vi "数据查询_数据查询.vi"() -> ()   [LabVIEW 2016, in "数据查询.lvlib"]
uses:
  System.Windows.Forms
  <vilib>/Utility/miscctls.llb/LVPointTypeDef.ctl
  <userlib>/_OpenG.lib/array/array.llb/Sort 2D Array (String)__ogtk.vi
  <vilib>/ptbypt/NI_PtbyPt.lvlib
panel:
  in  "数据类型":string(combo)="N"
  out "columns":string[](array[string])
  out "表格":string[][](table)
  in  "剔除异常数据":bool=TRUE
  in  "WebBrowser":refnum<k24>(container)
  in  "列表框":i32(listbox)
  in  "导出":bool
  in  "测量模式":string(combo)="全部数据"
  out "选中数据表":string
  in  "查询":bool
  in  "结束日期":string="2050/01/01"
  in  "起始日期":string="2010/01/01"
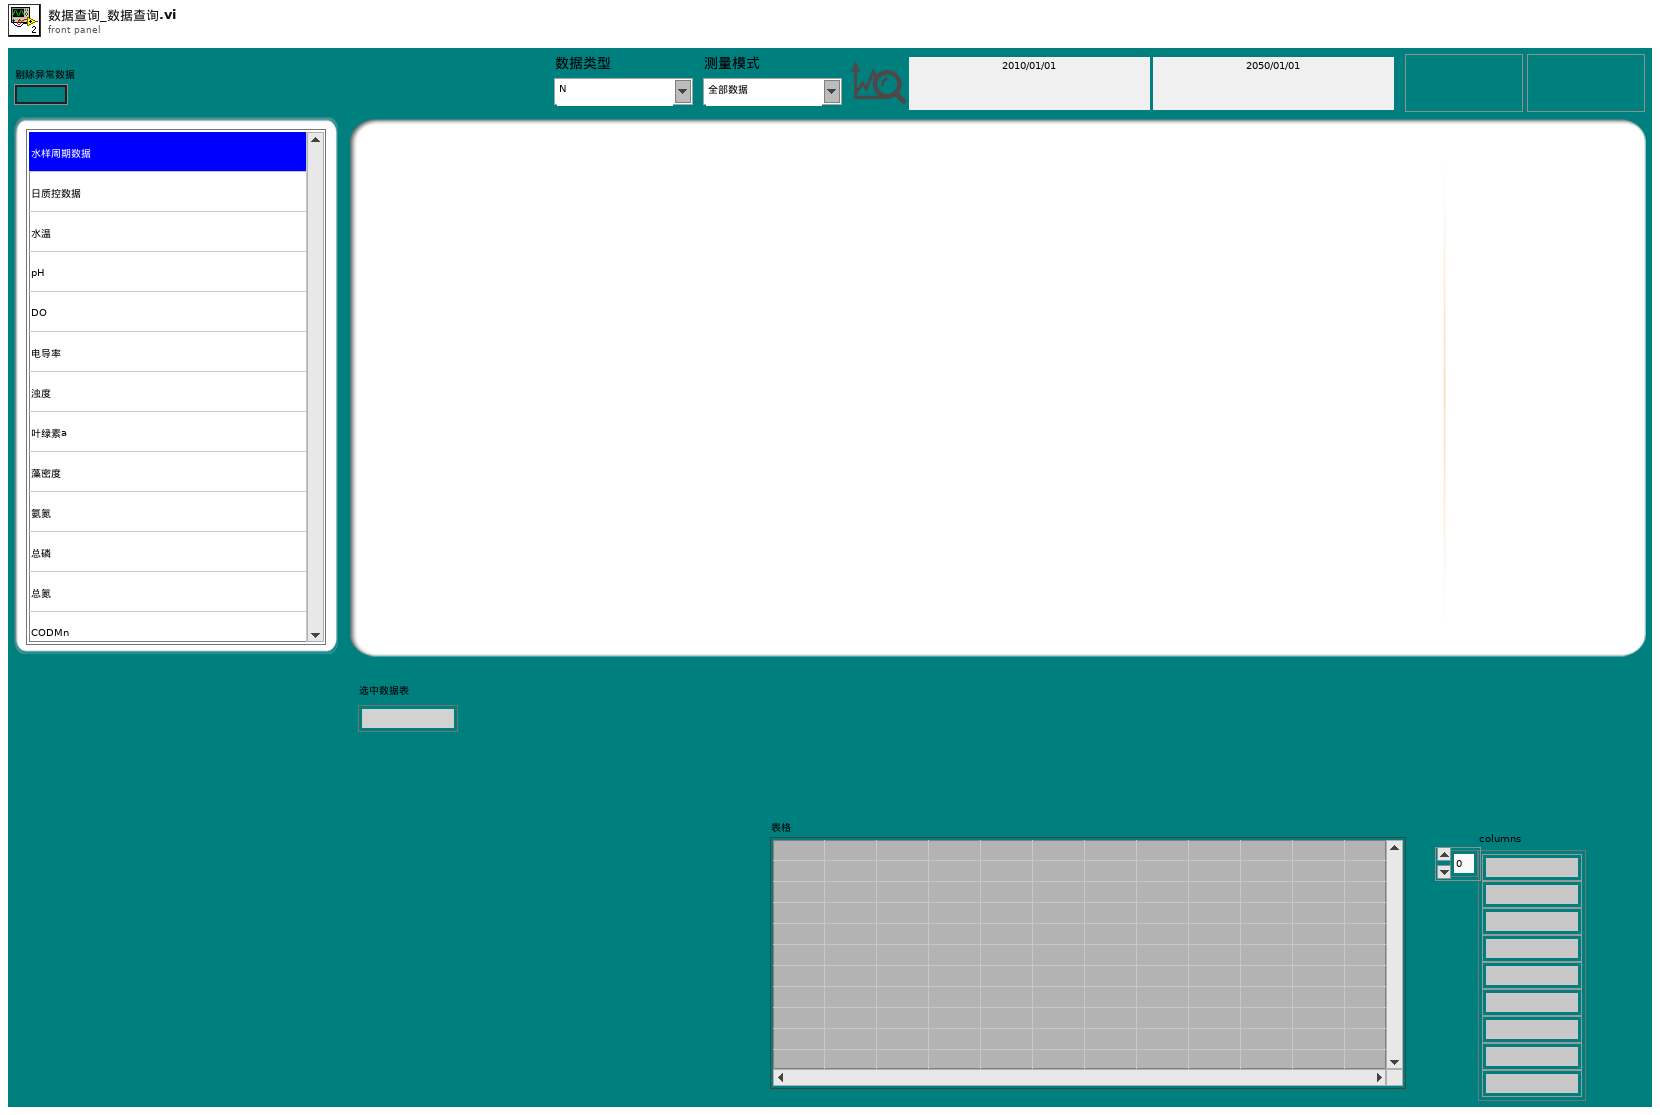
[diagram p1: front panel]
types:
  T1 = typedef "LVPointTypeDef.ctl" = cluster{"Horizontal":i16, "Vertical":i16}
  T2 = typedef "LVDateTimeRec.ctl" = cluster{"秒数的小数部分":dbl, "秒":i32, "分":i32, "时":i32, "日":i32, "月":i32, "年":i32, "天数（周）":i32, "天数（年）":i32, "DST":i32}
  T3 = typedef "数据查询.lvlib/数据查询单选控件.ctl" = enum32{"数据查询", "仪器数据", "仪器日志", "报警信息", "校准日志"}
  T4 = typedef "Rendezvous RefNum" = refnum<k1>
  T5 = enum8{"Enabled", "Disabled", "Disabled and Grayed Out"}
  T6 = typedef "数据库类型.ctl" = enum16{"Access", "SQLite"}
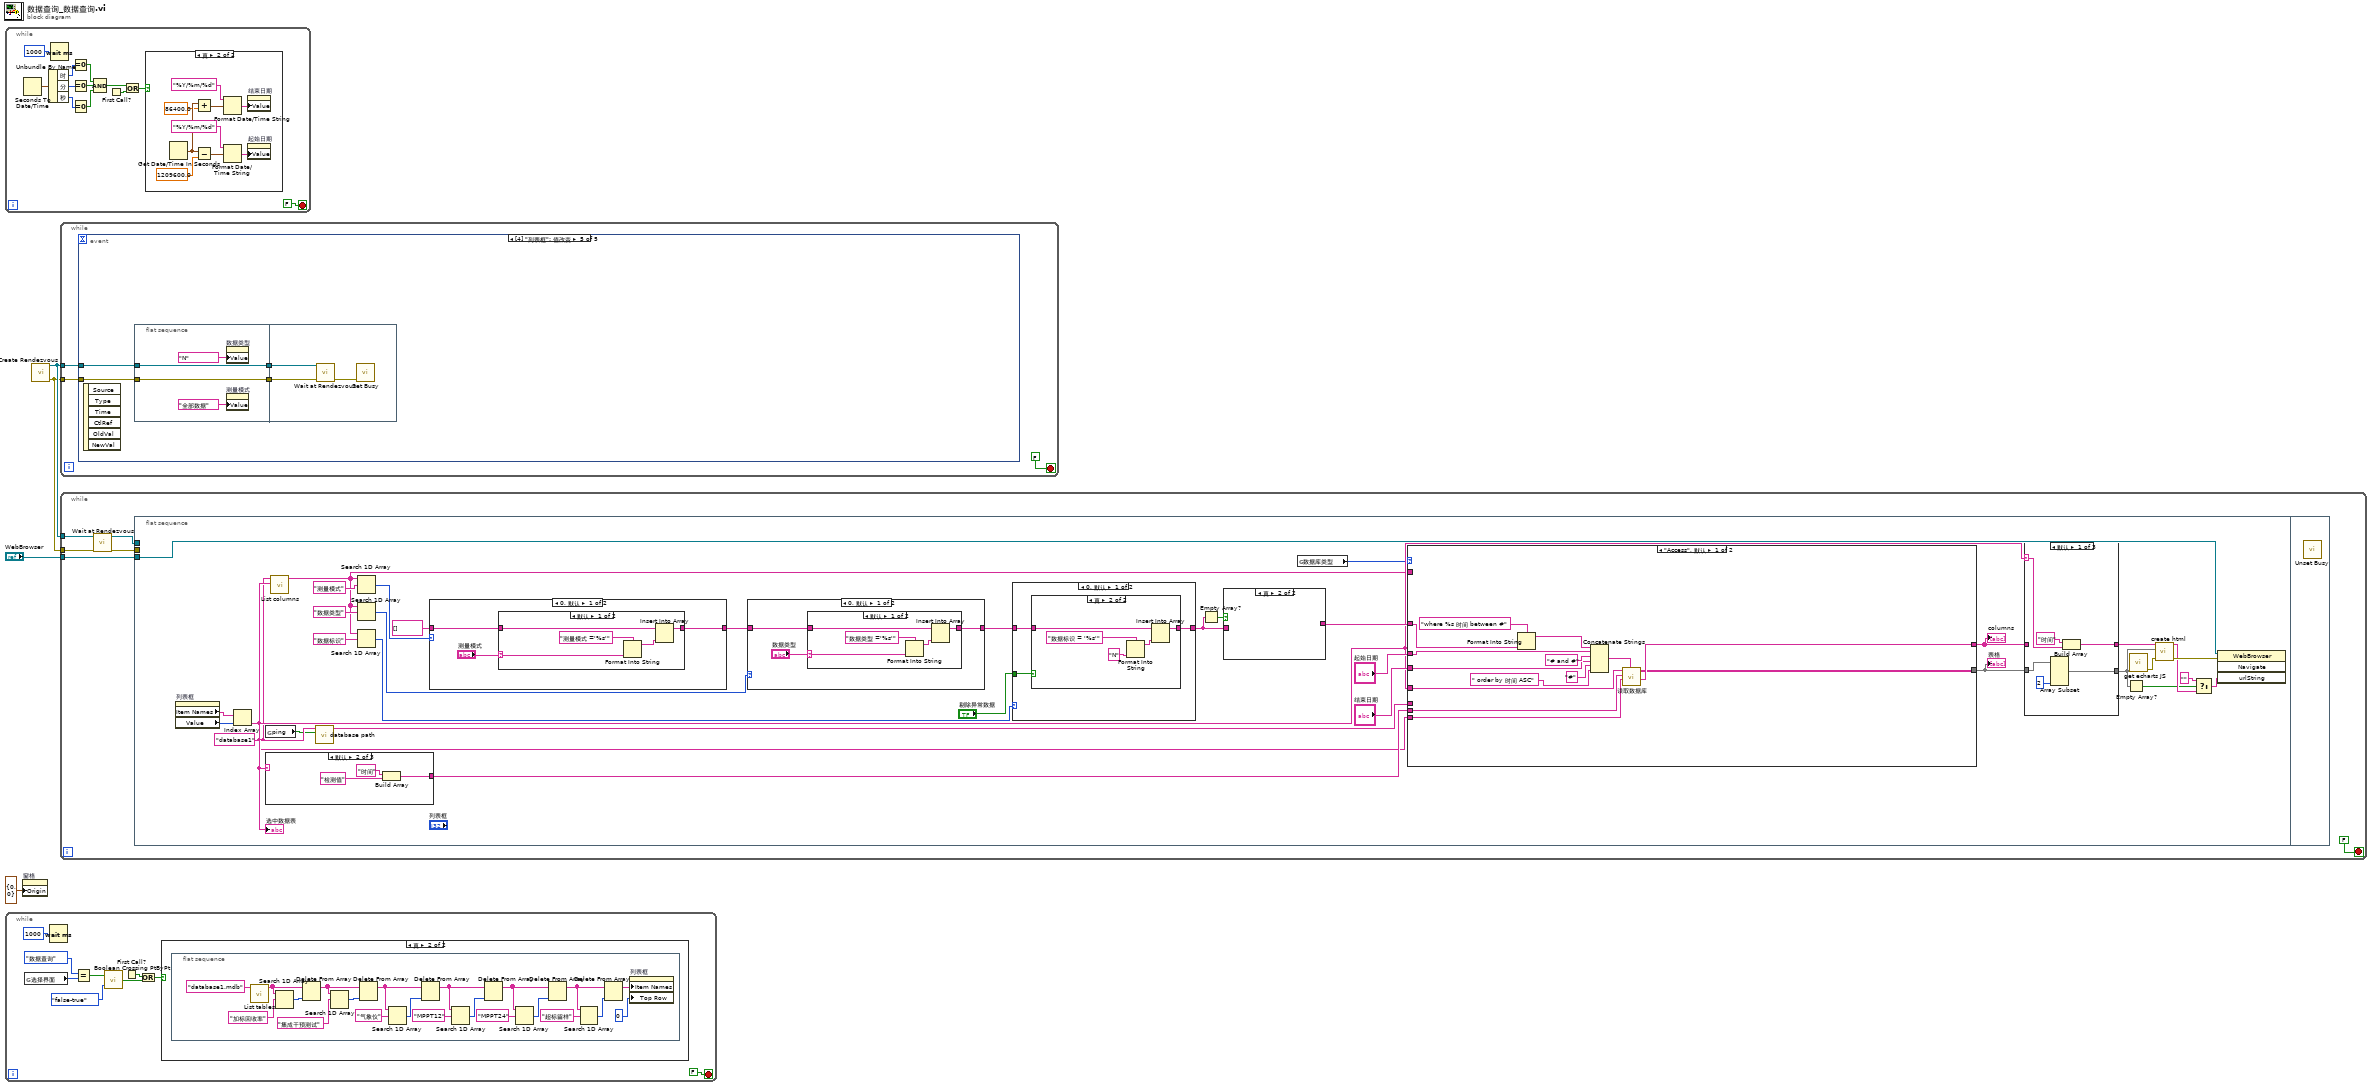
[diagram p0: block diagram]
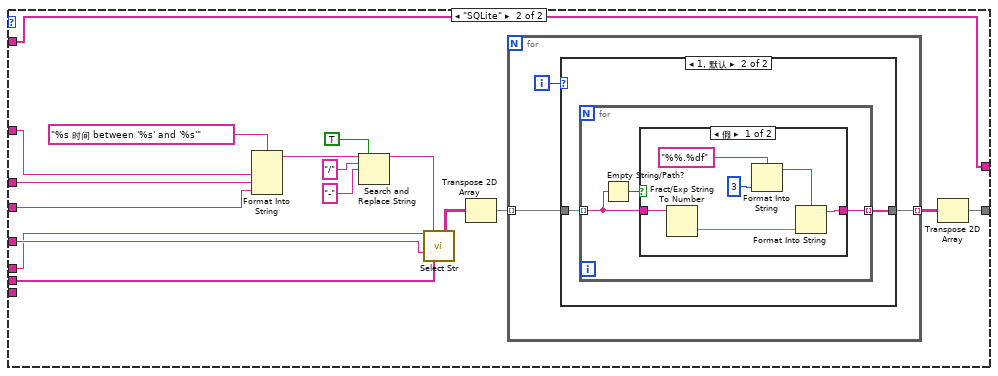
[diagram p3: hidden frame]
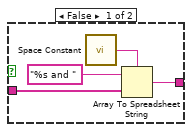
[diagram p6: hidden frame]
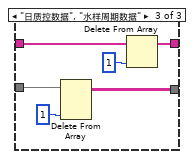
[diagram p14: hidden frame]
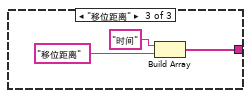
[diagram p16: hidden frame]
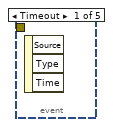
[diagram p18: hidden frame]
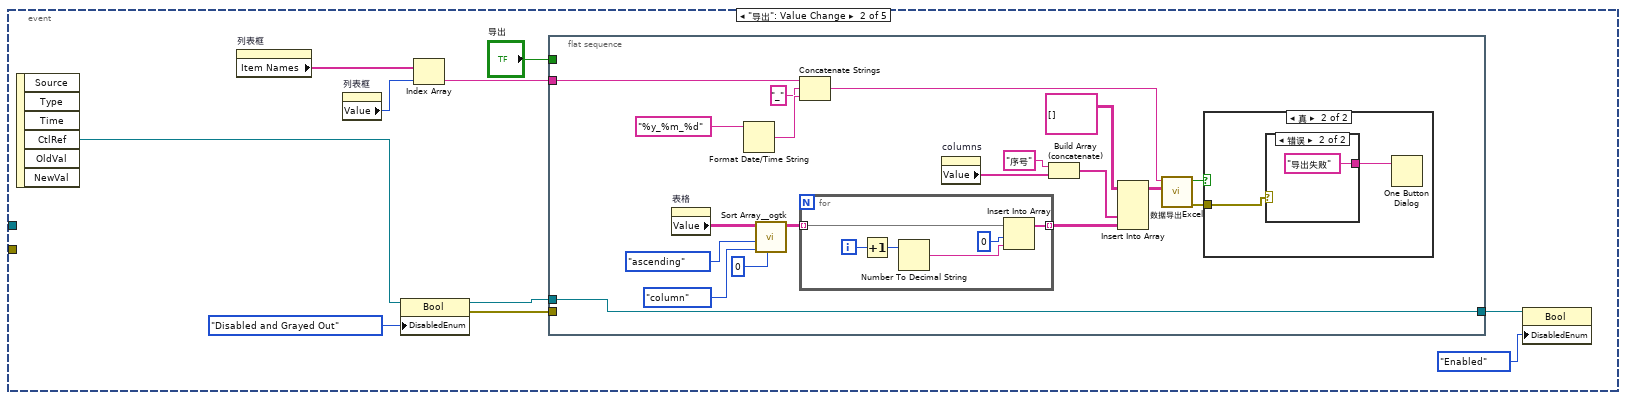
[diagram p19: hidden frame]
diagram:
  n1 = while {
    stop <- FALSE stop-if-true
    n2 = Seconds To Date/Time() -> (date time rec=w16:T2)  [unwired: 2 in]
    n3 = Unbundle By Name(w16) -> ("时"=w15:i32, "分"=w14:i32, "秒"=w13:i32)
    n4 = Wait (ms)(milliseconds to wait=u32 1000 ("等待时间（毫秒）")) -> ()  [unwired: 1 out]
    n5 = Equal To 0?(x=w15) -> (x = 0?=w12:bool)
    n6 = Equal To 0?(x=w14) -> (x = 0?=w11:bool)
    n7 = Equal To 0?(x=w13) -> (x = 0?=w10:bool)
    n8 = Compound Arithmetic op=AND ("复合运算")(w12, w11, w10) -> (w7:bool)
    n9 = First Call?() -> (First Call?: T/F=w5:bool)
    n10 = Or(x=w7, y=w5) -> (x .or. y?=w6:bool)
    n11 = case shown="真" w6 {
      frame False {
      }
      frame True {
        n12 = Get Date/Time In Seconds() -> (seconds since 1Jan1904=w21:timestamp)
        n13 = Add(x=w21, y=86400.0) -> (x+y=w19:timestamp)
        n14 = Subtract(x=w21, y=1209600.0) -> (x-y=w22:timestamp)
        n15 = Format Date/Time String(time format string (%c)="%Y/%m/%d" ("时间格式字符串(%c)"), seconds (now)=w19) -> (date/time string=w18:string)  [unwired: 1 in]
        n16 = Format Date/Time String(time format string (%c)="%Y/%m/%d" ("时间格式字符串(%c)"), seconds (now)=w22) -> (date/time string=w24:string)  [unwired: 1 in]
        n17 = property on="结束日期" class="Str"("Value"=w18) -> ()  [unwired: 2 in, 2 out]
        n18 = property on="起始日期" class="Str"("Value"=w24) -> ()  [unwired: 2 in, 2 out]
      }
    }
  }
  n19 = while {
    stop <- FALSE stop-if-true
    n20 = global read "全局变量.vi" "选择界面"() -> (w32:T3)
    n21 = Wait (ms)(milliseconds to wait=u32 1000 ("等待时间（毫秒）")) -> ()  [unwired: 1 out]
    n22 = Equal?(x=数据查询单选控件."数据查询", y=w32) -> (x = y?=w30:bool)
    n23 = call <vilib>:"Boolean Crossing PtByPt.vi"("direction"=enum16{"either", "false-true", "true-false"}."false-true", "input"=w30) -> ("crossing"=w28:bool)  [unwired: 1 in]
    n24 = First Call?() -> (First Call?: T/F=w26:bool)
    n25 = Or(x=w26, y=w28) -> (x .or. y?=w27:bool)
    n26 = case shown="真" w27 {
      frame False {
      }
      frame True {
        n27 = flat-sequence {
          frame #0 {
            n28 = call "List tables.vi"("database"="database1.mdb") -> ("tables"=w39:string[])  [unwired: 9 in, 1 out]
            n29 = Search 1D Array(1D array=w39, element="加标回收率" ("元素")) -> (index of element=w40:i32)  [unwired: 1 in]
            n30 = Delete From Array(array=w39, index=w40) -> (array with subset deleted=w42:string[])  [unwired: 1 in, 1 out]
            n31 = Search 1D Array(1D array=w42, element="集成干预测试" ("元素")) -> (index of element=w41:i32)  [unwired: 1 in]
            n32 = Delete From Array(array=w42, index=w41) -> (array with subset deleted=w45:string[])  [unwired: 1 in, 1 out]
            n33 = Search 1D Array(1D array=w45, element="气象仪" ("元素")) -> (index of element=w43:i32)  [unwired: 1 in]
            n34 = Delete From Array(array=w45, index=w43) -> (array with subset deleted=w48:string[])  [unwired: 1 in, 1 out]
            n35 = Search 1D Array(1D array=w48, element="MPPT12" ("元素")) -> (index of element=w47:i32)  [unwired: 1 in]
            n36 = Delete From Array(array=w48, index=w47) -> (array with subset deleted=w51:string[])  [unwired: 1 in, 1 out]
            n37 = Search 1D Array(1D array=w51, element="MPPT24" ("元素")) -> (index of element=w49:i32)  [unwired: 1 in]
            n38 = Delete From Array(array=w51, index=w49) -> (array with subset deleted=w52:string[])  [unwired: 1 in, 1 out]
            n39 = Search 1D Array(1D array=w52, element="超标留样" ("元素")) -> (index of element=w54:i32)  [unwired: 1 in]
            n40 = Delete From Array(array=w52, index=w54) -> (array with subset deleted=w55:string[])  [unwired: 1 in, 1 out]
            n41 = property on="列表框" class="LstBox (严格)"("Item Names"=w55, "Top Row"=0 ("顶行")) -> ()  [unwired: 2 in, 2 out]
          }
        }
      }
    }
  }
  n42 = property on="窗格" class="Pane"("Origin"=T1 {"Horizontal"=0, "Vertical"=0} ("原点")) -> ()  [unwired: 2 in, 2 out]
  n43 = call <vilib>:"Create Rendezvous.vi"() -> ("error out"=w1:errorcluster, "rendezvous"=w2:T4)  [unwired: 5 in, 1 out]
  n44 = while {
    tunnel: w2 -> [w57]
    tunnel: w1 -> [w56]
    stop <- FALSE stop-if-true
    n45 = event shown="[4] \"列表框\": 值改变" {
      selector: _ -> [_ _ _ _ _]
      dyn-events: _ -> [_ _ _ _ _]
      timeout: _ -> [_ _ _ _ _]
      tunnel: w57 -> [_ _ _ w104 w107]
      tunnel: w56 -> [_ _ _ w103 w105]
      event Timeout {
        n46 = event-data() -> ()  [unwired: 1 in, 3 out]
      }
      event "导出": Value Change {
        n47 = event-data() -> ("CtlRef"=w68:refnum<vi>)  [unwired: 1 in, 5 out]
        n48 = property on="列表框" class="LstBox (严格)"() -> ("Item Names"=w61:string[])  [unwired: 2 in, 2 out]
        n49 = property on="列表框" class="LstBox (严格)"() -> ("Value"=w60:i32)  [unwired: 2 in, 2 out]
        n50 = property class="Bool"(reference=w68, "DisabledEnum"=T5."Disabled and Grayed Out" ("禁用")) -> (reference out=w65:refnum<vi>, error out=w66:errorcluster)  [unwired: 1 in]
        n51 = Index Array(array=w61, index=w60) -> (element=w59:string)
        n52 = flat-sequence {
          tunnel: w66 -> [_]
          tunnel: [w84] -> w64
          tunnel: w65 -> [w84]
          tunnel: "导出" -> [_]
          tunnel: w59 -> [w74]
          frame #0 {
            n53 = property on="表格" class="Tbl (严格)"() -> ("Value"=w70:string[][])  [unwired: 2 in, 2 out]
            n54 = Format Date/Time String(time format string (%c)="%y_%m_%d" ("时间格式字符串(%c)")) -> (date/time string=w81:string)  [unwired: 2 in]
            n55 = call-poly <userlib>:"Sort Array__ogtk.vi"("Column/Row to Sort By"=u32 0, "Sort By in"=enum16{"row", "column"}."column", "Order"=enum16{"ascending", "descending"}."ascending", "Array in"=w70) -> ("Sorted Array out"=w78:string[][])  [unwired: 4 in, 3 out]
            n56 = Concatenate Strings(w74, "_" ("字符串"), w81) -> (w79:string)
            n57 = for {
              tunnel: w78 -> [w96] mode=indexing
              tunnel: [w95] -> w71 mode=indexing
              i -> [w97]
              n58 = Increment(x=w97) -> (x+1=w93:i32)
              n59 = Number To Decimal String(number=w93) -> (decimal integer string=w92:string)  [unwired: 1 in]
              n60 = Insert Into Array(array=w96, index=0 ("索引"), new element=w92) -> (w95:string[])
            }
            n61 = property on="columns" class="Arr (严格)"() -> ("Value"=w69:string[])  [unwired: 2 in, 2 out]
            n62 = Build Array (concatenate)("序号" ("新元素/子数组"), w69) -> (w72:string[])
            n63 = Insert Into Array(array=string[][] [], new element #1=w72, new element #2=w71) -> (w77:string[][])  [unwired: 2 in]
            n64 = call "数据导出Excel.vi"("text data"=w77, "default name"=w79) -> ("error out"=w76:errorcluster, "布尔"=w75:bool)  [unwired: 8 in]
            n65 = case shown="真" w75 {
              tunnel: w76 -> [_ w89]
              frame False {
              }
              frame True {
                n66 = case shown="错误" w89 {
                  tunnel: ["导出成功" ("消息") "导出失败" ("消息")] -> w88
                  frame No Error {
                  }
                  frame Error {
                  }
                }
                n67 = One Button Dialog(message=w88) -> ()  [unwired: 1 in, 1 out]
              }
            }
          }
        }
        n68 = property class="Bool"(reference=w64, "DisabledEnum"=T5."Enabled" ("禁用")) -> ()  [unwired: 1 in, 2 out]
      }
      event "起始日期", "结束日期": Mouse Down {
        n69 = event-data() -> ("CtlRef"=w101:refnum<vi>)  [unwired: 1 in, 7 out]
        n70 = property class="Str"(reference=w101) -> (reference out=w99:refnum<vi>, "Value"=w100:string)  [unwired: 1 in, 1 out]
        n71 = call "日期键盘.vi"("原值"=w100) -> ("x+y"=w98:string)  [unwired: 10 in]
        n72 = property class="Str"(reference=w99, "Val(Sgnl)"=w98) -> ()  [unwired: 1 in, 2 out]
      }
      event "查询", "起始日期", "结束日期", "测量模式", "剔除异常数据", "数据类型": Value Change {
        n73 = event-data() -> ()  [unwired: 1 in, 6 out]
        n74 = call <vilib>:"Wait at Rendezvous.vi"("error in (no error)"=w103, "rendezvous"=w104) -> ("error out"=w102:errorcluster)  [unwired: 3 in, 2 out]
        n75 = call <vilib>:"Set Busy.vi"("error in (no error)"=w102) -> ()  [unwired: 9 in, 2 out]
      }
      event "列表框": Value Change {
        n76 = event-data() -> ()  [unwired: 1 in, 6 out]
        n77 = flat-sequence {
          tunnel: [w110] -> w108
          tunnel: w107 -> [w110]
          tunnel: [w109] -> w106
          tunnel: w105 -> [w109]
          tunnel: w108 -> [w115]
          tunnel: w106 -> [w114]
          frame #0 {
            n78 = property on="数据类型" class="CmbBox"("Value"="N" ("数据类型")) -> ()  [unwired: 2 in, 2 out]
            n79 = property on="测量模式" class="CmbBox"("Value"="全部数据" ("测量模式")) -> ()  [unwired: 2 in, 2 out]
          }
          frame #1 {
            n80 = call <vilib>:"Wait at Rendezvous.vi"("error in (no error)"=w114, "rendezvous"=w115) -> ("error out"=w113:errorcluster)  [unwired: 3 in, 2 out]
            n81 = call <vilib>:"Set Busy.vi"("error in (no error)"=w113) -> ()  [unwired: 9 in, 2 out]
          }
        }
      }
    }
  }
  n82 = while {
    tunnel: "WebBrowser" -> [w120]
    tunnel: w2 -> [w119]
    tunnel: w1 -> [w118]
    stop <- FALSE stop-if-true
    n83 = call <vilib>:"Wait at Rendezvous.vi"("error in (no error)"=w118, "rendezvous"=w119) -> ("error out"=w117:errorcluster, "rendezvous out"=w116:T4)  [unwired: 3 in, 1 out]
    n84 = flat-sequence {
      tunnel: w120 -> [w154]
      tunnel: w117 -> [_]
      tunnel: w116 -> [_]
      frame #0 {
        w124 = "database1" ("database")
        n85 = property on="列表框" class="LstBox (严格)"() -> ("Item Names"=w146:string[], "Value"=w145:i32)  [unwired: 2 in, 2 out]
        n86 = Index Array(array=w146, index=w145) -> (element=w137:string)
        "选中数据表" <- w137
        n87 = global read "全局变量.vi" "ping"() -> (w123:bool)
        n88 = case shown="默认" w137 {
          tunnel: [_ w252 w255] -> w148
          frame "多参数", "环境参数", "日质控数据", "水样周期数据" {
          }
          frame Default {
            n89 = Build Array("时间", "检测值") -> (w252:string[])
          }
          frame "移位距离" {
            n90 = Build Array("时间", "移位距离") -> (w255:string[])
          }
        }
        n91 = call "List columns.vi"("table"=w137, "database"=w124) -> ("columns"=w126:string[])  [unwired: 8 in, 1 out]
        n92 = call "database path.vi"("ping"=w123, "database"=w124) -> ("Path out"=w125:string)  [unwired: 8 in, 1 out]
        n93 = Search 1D Array(1D array=w126, element="测量模式" ("元素")) -> (index of element=w132:i32)  [unwired: 1 in]
        n94 = Search 1D Array(1D array=w126, element="数据类型" ("元素")) -> (index of element=w130:i32)  [unwired: 1 in]
        n95 = Search 1D Array(1D array=w126, element="数据标识" ("元素")) -> (index of element=w129:i32)  [unwired: 1 in]
        n96 = case shown="0, 默认" w132 {
          tunnel: string[] [] -> [w230 w237]
          tunnel: [w228 w237] -> w131
          frame 0, Default {
            n97 = case shown="默认" "测量模式" {
              selector: "测量模式" -> [w231 _]
              tunnel: w230 -> [w234 w236]
              tunnel: [w232 w236] -> w228
              frame Default {
                n98 = Format Into String(format string="测量模式 ='%s'" ("condition"), w231) -> (resulting string=w233:string)  [unwired: 2 in, 1 out]
                n99 = Insert Into Array(array=w234, new element=w233) -> (w232:string[])  [unwired: 1 in]
              }
              frame "全部数据" {
              }
            }
          }
          frame -1 {
          }
        }
        n100 = case shown="0, 默认" w130 {
          tunnel: [w219 w227] -> w133
          tunnel: w131 -> [w218 w227]
          frame 0, Default {
            n101 = case shown="默认" "数据类型" {
              selector: "数据类型" -> [w221 _]
              tunnel: w218 -> [w224 w226]
              tunnel: [w222 w226] -> w219
              frame Default {
                n102 = Format Into String(format string="数据类型 ='%s'" ("condition"), w221) -> (resulting string=w223:string)  [unwired: 2 in, 1 out]
                n103 = Insert Into Array(array=w224, new element=w223) -> (w222:string[])  [unwired: 1 in]
              }
              frame "全部数据" {
              }
            }
          }
          frame -1 {
          }
        }
        n104 = case shown="0, 默认" w129 {
          tunnel: "剔除异常数据" -> [w210 _]
          tunnel: [w209 w217] -> w128
          tunnel: w133 -> [w208 w217]
          frame 0, Default {
            n105 = case shown="真" w210 {
              tunnel: w208 -> [w211 w216]
              tunnel: [w211 w215] -> w209
              frame False {
              }
              frame True {
                n106 = Format Into String(format string="数据标识 = '%s'" ("condition"), "N" ("String")) -> (resulting string=w212:string)  [unwired: 2 in, 1 out]
                n107 = Insert Into Array(array=w216, new element=w212) -> (w215:string[])  [unwired: 1 in]
              }
            }
          }
          frame -1 {
          }
        }
        n108 = Empty Array?(array=w128) -> (empty?=w127:bool)
        n109 = case shown="真" w127 {
          tunnel: [w207 _] -> w138
          tunnel: w128 -> [w204 _]
          frame False {
            n110 = call <vilib>:"Space Constant.vi"() -> ("String"=w206:string)
            n111 = Array To Spreadsheet String(delimiter (Tab)=w206, array=w204, 3:"%s and " ("格式字符串")) -> (spreadsheet string=w207:string)
          }
          frame True {
          }
        }
        n112 = global read "外部调用接口全局变量.vi" "数据库类型"() -> (w122:T6)
        n113 = case shown="\"Access\", 默认" w122 {
          tunnel: "结束日期" -> [w166 w178]
          tunnel: "起始日期" -> [w165 w179]
          tunnel: [w164 w176] -> w151
          tunnel: [w163 w177] -> w149
          tunnel: w148 -> [w162 w172]
          tunnel: w138 -> [w161 w180]
          tunnel: w137 -> [w158 w173]
          tunnel: w126 -> [_ w176]
          tunnel: w125 -> [_ w171]
          tunnel: w124 -> [w157 _]
          frame "Access", Default {
            n114 = Format Into String(format string="where %s 时间 between #" ("condition"), w161) -> (resulting string=w159:string)  [unwired: 2 in, 1 out]
            n115 = Concatenate Strings(w159, w165, "# and #" ("condition"), w166, "#" ("condition"), " order by 时间 ASC" ("字符串")) -> (w170:string)
            n116 = call "读取数据库.vi"("condition"=w170, "database"=w157, "显示项"=w162, "组合框"=w158) -> ("columns"=w164:string[], "表格"=w163:string[][])  [unwired: 4 in, 2 out]
          }
          frame "SQLite" {
            n117 = Format Into String(format string="%s 时间 between '%s' and '%s'" ("格式字符串"), w180, w179, w178) -> (resulting string=w183:string)  [unwired: 2 in, 1 out]
            n118 = Search and Replace String(replace all?=TRUE ("替换全部？(F)"), input string=w183, search string="/" ("搜索字符串"), replace string="-" ("替换字符串(\"\")")) -> (result string=w175:string)  [unwired: 4 in, 3 out]
            n119 = call "Select Str.vi"("DB Path"=w171, "Where Clause"=w175, "Tables Name"=w173, "Columns"=w172) -> ("Results"=w174:string[][])  [unwired: 8 in, 3 out]
            n120 = Transpose 2D Array(2D array=w174) -> (transposed array=w182:string[][])
            n121 = for {
              tunnel: w182 -> [w190] mode=indexing
              tunnel: [w189] -> w181 mode=indexing
              i -> [w188]
              n122 = case shown="1, 默认" w188 {
                tunnel: w190 -> [w191 w193]
                tunnel: [w191 w192] -> w189
                frame 0 {
                }
                frame 1, Default {
                  n123 = for {
                    tunnel: w193 -> [w195] mode=indexing
                    tunnel: [w196] -> w192 mode=indexing
                    n124 = Empty String/Path?(string/path=w195) -> (empty?=w194:bool)
                    n125 = case shown="假" w194 {
                      tunnel: [w200 w203] -> w196
                      tunnel: w195 -> [w197 w203]
                      frame False {
                        n126 = Fract/Exp String To Number(string=w197) -> (number=w199:dbl)  [unwired: 3 in, 1 out]
                        n127 = Format Into String(format string="%%.%df" ("格式字符串"), 3 ("输入 1")) -> (resulting string=w202:string)  [unwired: 2 in, 1 out]
                        n128 = Format Into String(format string=w202, w199) -> (resulting string=w200:string)  [unwired: 2 in, 1 out]
                      }
                      frame True {
                      }
                    }
                  }
                }
              }
            }
            n129 = Transpose 2D Array(2D array=w181) -> (transposed array=w177:string[][])
          }
        }
        "表格" <- w149
        "columns" <- w151
        n130 = case shown="默认" w137 {
          selector: w137 -> [w240 _ _]
          tunnel: w151 -> [_ w245 w251]
          tunnel: [w239 w245 w250] -> w150
          tunnel: w149 -> [w243 w244 w248]
          tunnel: [w242 w244 w247] -> w141
          frame Default {
            n131 = Array Subset(array=w243, length (col)=2 ("长度")) -> (w242:string[][])  [unwired: 3 in]
            n132 = Build Array("时间", w240) -> (w239:string[])
          }
          frame "多参数", "环境参数" {
          }
          frame "日质控数据", "水样周期数据" {
            n133 = Delete From Array(array=w248, index (col)=1 ("禁用的索引 (列)")) -> (array with subset deleted=w247:string[][])  [unwired: 2 in, 1 out]
            n134 = Delete From Array(array=w251, index=1 ("索引")) -> (array with subset deleted=w250:string[])  [unwired: 1 in, 1 out]
          }
        }
        n135 = Empty Array?(array=w141) -> (empty?=w140:bool)
        n136 = call "get echarts JS.vi"() -> ("error out"=w153:errorcluster)  [unwired: 11 in]
        n137 = call "create html.vi"("error in (no error)"=w153, "data"=w141, "columns"=w150) -> ("error out"=w152:errorcluster, "url"=w144:string)  [unwired: 7 in]
        n138 = Select(t="", s=w140, f=w144) -> (s? t:f=w143:string)
        n139 = invoke class="WebBrowser" method="Navigate"(reference=w154, error in=w152, "urlString"=w143) -> ()  [unwired: 1 in, 4 out]
      }
      frame #1 {
        n140 = call <vilib>:"Unset Busy.vi"() -> ()  [unwired: 11 in, 1 out]
      }
    }
  }
